vi "Drive Train Global.vi"() -> ()   [LabVIEW 2018]
panel:
  out "Wheel Angles":T1
  in  "Rot. Point Y":dbl
  in  "Rot. Point X":dbl
  in  "Wheel Turn PID Values":T2
  in  "Z Command":dbl
  in  "Y Command":dbl
  out "Gyro Information":T3
  in  "X Command":dbl
  in  "Current State":enum16{"Reached Position", "Going to Position"}(ring)
  in  "Current Mode":T4(ring)
  out "Extra Info":bool
  out "Velocity":cluster{"X":dbl, "Y":dbl, "Z":dbl}
  out "Position":cluster{"X":dbl, "Y":dbl, "Z":dbl}
  out "Wheel Drive Encoders":T5
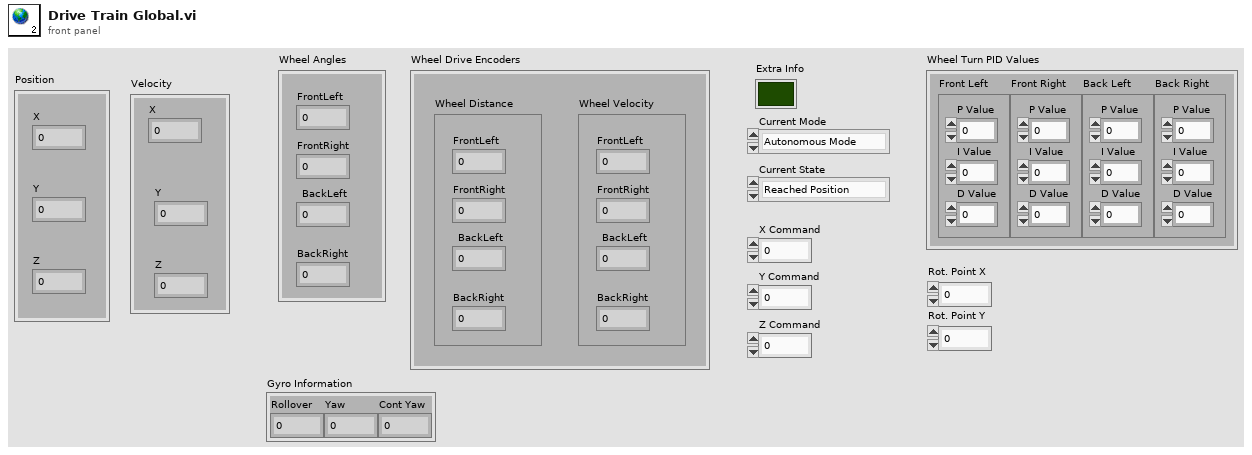
[diagram p1: front panel]
types:
  T1 = cluster{"FrontLeft":dbl, "FrontRight":dbl, "BackLeft":dbl, "BackRight":dbl}
  T2 = cluster{"Front Left":cluster{"P Value":dbl, "I Value":dbl, "D Value":dbl}, "Front Right":cluster{"P Value":dbl, "I Value":dbl, "D Value":dbl}, "Back Left":cluster{"P Value":dbl, "I Value":dbl, "D Value":dbl}, "Back Right":cluster{"P Value":dbl, "I Value":dbl, "D Value":dbl}}
  T3 = cluster{"Rollover":dbl, "Yaw":dbl, "Cont Yaw":dbl}
  T4 = enum16{"Autonomous Mode", "Field Oriented", "Robot Oriented", "Tank Mode"}
  T5 = cluster{"Wheel Velocity":cluster{"FrontLeft":dbl, "FrontRight":dbl, "BackLeft":dbl, "BackRight":dbl}, "Wheel Distance":cluster{"FrontLeft":dbl, "FrontRight":dbl, "BackLeft":dbl, "BackRight":dbl}}
diagram:
